vi "Labview Receiver ClientI#1.vi"() -> ()   [LabVIEW 2020]
panel:
  in  "stop":bool
  out "mode (standard)":T1(ring)
  out "Received Data":dbl[](array[numeric]) format="%#_18g"
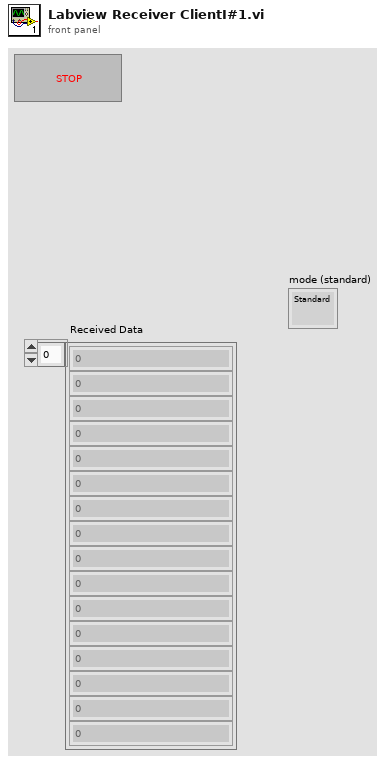
[diagram p1: front panel]
types:
  T1 = enum16{"Standard", "Buffered", "CRLF", "Immediate"}
  T2 = cluster{"Client#":string, "Status":string, "VarFunction":dbl}
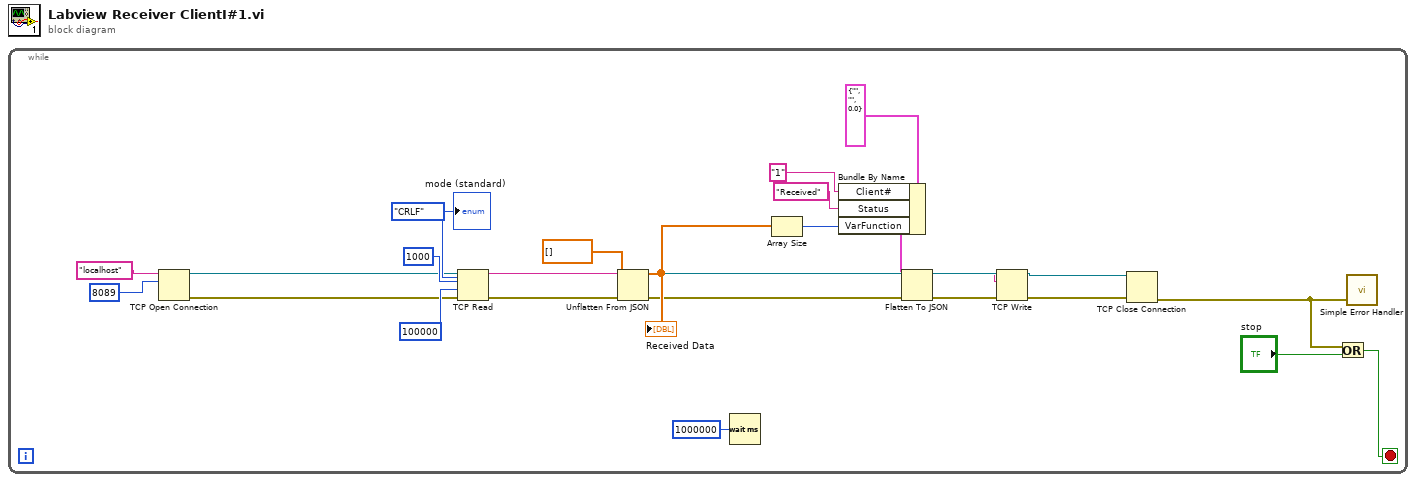
[diagram p0: block diagram]
diagram:
  n1 = while {
    stop <- w25 stop-if-true
    w24 = T1."CRLF" ("mode (standard)")
    n2 = TCP Open Connection(address="localhost", remote port or service name=8089) -> (connection ID=w7:refnum<k5>, error out=w6:errorcluster)  [unwired: 3 in]
    n3 = TCP Read(connection ID=w7, bytes to read=1000, error in (no error)=w6, 7:w24, 9:100000 ("timeout ms (25000)")) -> (connection ID out=w17:refnum<k5>, data out=w23:string, error out=w18:errorcluster)
    n4 = Unflatten From JSON(JSON string=w23, type and defaults=dbl[] [], error in (no error)=w18) -> (value=w19:dbl[], error out=w16:errorcluster)  [unwired: 4 in]
    "Received Data" <- w19
    n5 = Wait (ms)(milliseconds to wait=u32 1000000) -> ()  [unwired: 1 out]
    n6 = Array Size(array=w19) -> (size(s)=w13:i32)
    n7 = Bundle By Name(cluster=T2 {"Client#"="", "Status"="", "VarFunction"=0.0}, "Client#"="1", "Status"="Received", "VarFunction"=w13) -> (w10:T2)
    n8 = Flatten To JSON(anything=w10, error in (no error)=w16) -> (JSON string=w14:string, 11:w15:errorcluster)  [unwired: 1 in]
    n9 = TCP Write(connection ID=w17, data in=w14, error in (no error)=w15) -> (connection ID out=w3:refnum<k5>, error out=w5:errorcluster)  [unwired: 1 in, 1 out]
    n10 = TCP Close Connection(connection ID=w3, error in (no error)=w5) -> (error out=w26:errorcluster)  [unwired: 1 in, 1 out]
    n11 = Or(x=w26, y="stop") -> (x .or. y?=w25:bool)
    n12 = call <vilib>:"Simple Error Handler.vi"("error in (no error)"=w26) -> ()  [unwired: 4 in, 5 out]
    "mode (standard)" <- w24
  }
